vi "CIMAQ_MaxMin.vi"(8 "error in (no error)":errorcluster, 11 "Img In":T1) -> (0 "error out":errorcluster, 2 "Minimal Value":sgl, 3 "Maximal Value":sgl)   [LabVIEW 2017]
uses:
  <vilib>/vision/Image Controls.llb/IMAQ Image.ctl
  <vilib>/vision/NI_Vision_Development_Module.lvlib
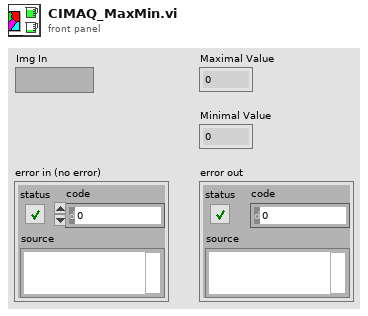
[diagram p1: front panel]
types:
  T1 = typedef "IMAQ Image.ctl" = refnum<image>
  T2 = cluster{"histogram":u32[], "Minimal Value":sgl, "Maximal Value":sgl, "Starting Value":sgl, "Interval Width":sgl, "Mean Value":sgl, "Standard  Variation":sgl, "Area (pixels)":i32}
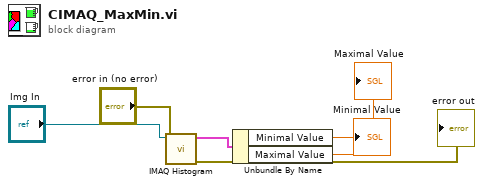
[diagram p0: block diagram]
diagram:
  n1 = call "IMAQ Histogram"("error in (no error)"="error in (no error)", "Image"="Img In") -> ("error out"=→"error out":errorcluster, "Histogram Report"=w2:T2)  [unwired: 8 in]
  n2 = Unbundle By Name(w2) -> ("Minimal Value"=→"Minimal Value":sgl, "Maximal Value"=→"Maximal Value":sgl)
